vi "go_to_next_line.vi"(8 "error in (no error)":errorcluster, 10 "Message_command in":T2={"No. of command"=3, "Parameters"=["2.31", "s"], "Address"="", "Boolean"=TRUE, "No. of line"=3, "Initial Time"=timestamp(3642518447.490892 s since 1904-01-01), "Current Time"=timestamp(0 s since 1904-01-01), "Status"="Stop DAQ...", "Sequence Ref."=refnum, "Temp check"=0, "Sequence_History"="", "Subsequence"=[]}, 11 "Command Queue in":T1) -> (0 "error out":errorcluster, 3 "Command Queue out":T1)   [LabVIEW 2020]
uses:
  Command_Message.ctl
  Command_Queue.ctl
panel:
  out "concatenated string":string="2:40 PM\tStop DAQ..."
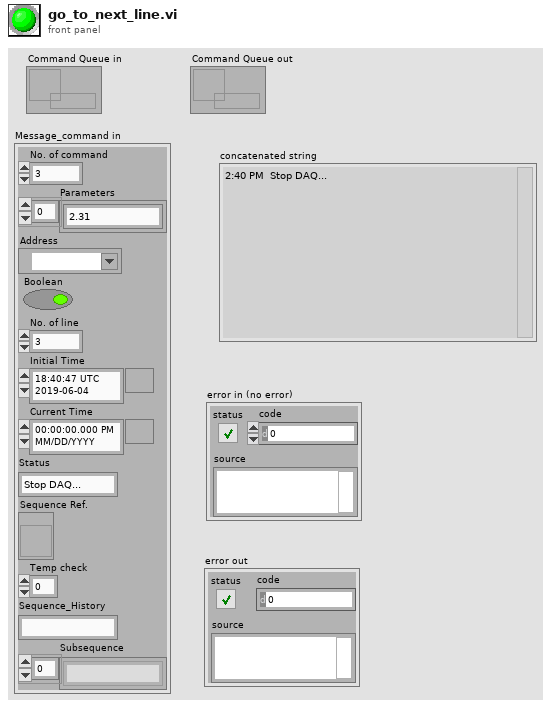
[diagram p1: front panel]
types:
  T1 = typedef "Command_Queue.ctl" = refnum<queue>
  T2 = typedef "Command_Message.ctl" = cluster{"No. of command":i32, "Parameters":string[], "Address":refnum<visa-resource-name>, "Boolean":bool, "No. of line":i32, "Initial Time":timestamp, "Current Time":timestamp, "Status":string, "Sequence Ref.":refnum<vi>, "Temp check":i32, "Sequence_History":string, "Subsequence":string[]}
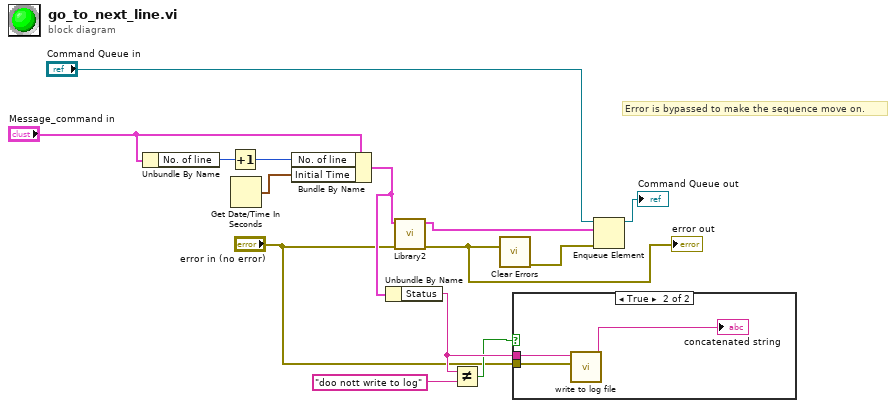
[diagram p0: block diagram]
diagram:
  # "Error is bypassed to make the sequence move on."
  n1 = Unbundle By Name("Message_command in") -> ("No. of line"=w10:i32)
  n2 = Increment(x=w10) -> (x+1=w13:i32)
  n3 = Get Date/Time In Seconds() -> (seconds since 1Jan1904=w14:timestamp)
  n4 = Bundle By Name(cluster="Message_command in", "No. of line"=w13, "Initial Time"=w14) -> (w7:T2)
  n5 = Unbundle By Name(w7) -> ("Status"=w6:string)
  n6 = call "Library2.vi"("Message_command_in"=w7, "error in (no error)"="error in (no error)") -> ("Message_command out"=w8:T2, "error out"=w1:errorcluster)  [unwired: 7 in]
  "error out" <- w1
  n7 = Not Equal?(x=w6, y="doo nott write to log") -> (x != y?=w4:bool)
  n8 = call <vilib>:"Clear Errors.vi"("error in (no error)"=w1) -> ("error out"=w2:errorcluster)  [unwired: 5 in, 1 out]
  n9 = case shown="True" w4 {
    tunnel: w6 -> [_ w17]
    tunnel: "error in (no error)" -> [_ w15]
    frame False {
    }
    frame True {
      n10 = call "write to log file.vi"("input"=w17, "error in"=w15) -> ("log"=→"concatenated string":string)  [unwired: 8 in]
    }
  }
  n11 = Enqueue Element(queue="Command Queue in", element=w8, error in (no error)=w2) -> (queue out=→"Command Queue out":T1)  [unwired: 1 in, 2 out]
